vi "PPMS.Close.vi"(8 "error in (no error)":errorcluster, 11 "instrument.PPMS in":refnum<class "instrument.PPMS.lvclass">) -> (0 "error out":errorcluster, 3 "instrument.PPMS out":refnum<class "instrument.PPMS.lvclass">)   [LabVIEW 2019, in "instrument.PPMS.lvclass"]
uses:
  instrument.PPMS.lvclass
  instrument.PPMS.lvclass/instrument.PPMS.ctl
  C:/Users/patrick/Documents/GitHub/levylabpitt/PPMS-Monitor-and-Control/lvsrc/drivers/QDInstrument_LabView/QDInstrument.dll
  drivers/QDInstrument_LabView/QDInstrument.dll
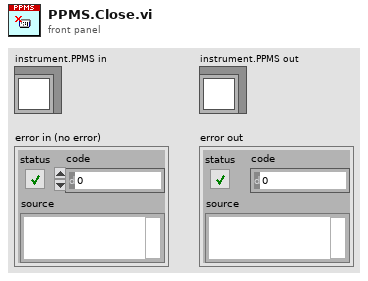
[diagram p1: front panel]
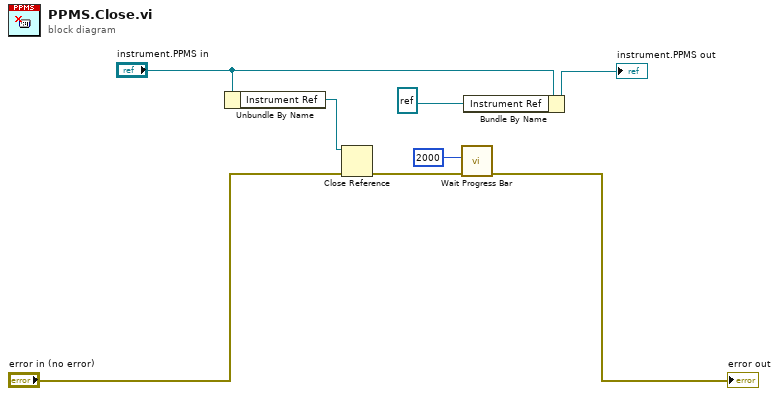
[diagram p0: block diagram]
diagram:
  n1 = Unbundle By Name("instrument.PPMS in") -> ("Instrument Ref"=w4:refnum<k24>)
  n2 = Close Reference(reference=w4, error in (no error)="error in (no error)") -> (error out=w3:errorcluster)
  n3 = call "Wait Progress Bar.vi"("error in (no error)"=w3, "wait (ms)"=u32 2000 ("milliseconds to wait")) -> ("error out"=→"error out":errorcluster)  [unwired: 9 in]
  n4 = Bundle By Name(cluster="instrument.PPMS in", "Instrument Ref"=refnum<k24> refnum) -> (→"instrument.PPMS out":refnum<class "instrument.PPMS.lvclass">)
